vi "Velocity_to_Drag.vi"(1 "Velocity":dbl) -> (0 "Drag":dbl)   [LabVIEW 2009]
uses:
  <vilib>/gmath/NI_Gmath.lvlib
panel:
  in  "Drag / Forward Velocity":cluster{"F":dbl, "V":dbl}[](array[cluster])=[{"F"=0.0, "V"=0.0}]
  # "Drag is in N\nVelocity in m/s"
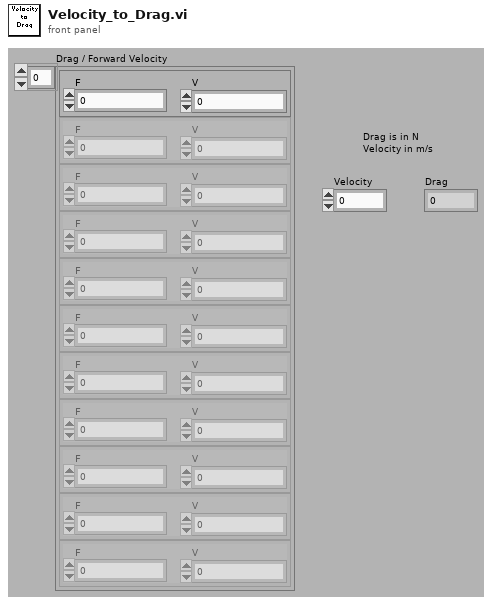
[diagram p1: front panel]
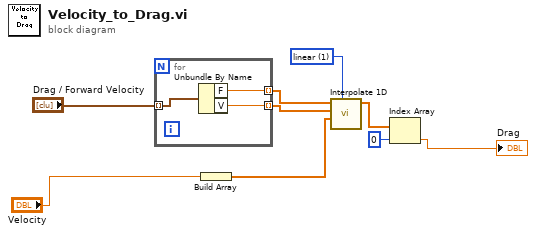
[diagram p0: block diagram]
diagram:
  w9 = 1 items=["nearest", "linear", "spline", "cubic Hermite", "Lagrange"] ("method")
  n1 = for {
    tunnel: "Drag / Forward Velocity" -> [w12] mode=indexing
    tunnel: [w11] -> w7 mode=indexing
    tunnel: [w10] -> w6 mode=indexing
    n2 = Unbundle By Name(w12) -> ("F"=w11:dbl, "V"=w10:dbl)
  }
  n3 = Build Array("Velocity") -> (w1:dbl[])
  n4 = call <vilib>:"Interpolate 1D.vi"("method"=w9, "xi"=w1, "X"=w6, "Y"=w7) -> ("yi"=w5:dbl[])  [unwired: 5 in, 2 out]
  n5 = Index Array(array=w5, index=0) -> (element=→"Drag":dbl)
